vi "aquisicao.vi"(8 "Stop":bool, 9 "Number of Samples":i32=100, 10 "Sample Rate":dbl=1000.0, 11 "Physical Channel":tag="Dev1/ai0") -> (2 "Waveform Chart":waveform(dbl)(graph))   [LabVIEW 2019]
doc: "This example demonstrates how to continuously acquire buffered voltage measurements using a DAQmx device.\n\nFor instructions on how to connect your signals to the DAQ device, refer to your device documentation."
uses:
  <vilib>/Utility/error.llb/DialogType.ctl
  <vilib>/DAQmx/create/channels.llb/DAQmx Create Channel (AI-Voltage-Basic).vi
  <vilib>/DAQmx/configure/timing.llb/DAQmx Timing (Sample Clock).vi
  <vilib>/DAQmx/configure/task.llb/DAQmx Configure Logging (TDMS).vi
  <vilib>/DAQmx/miscellaneous.llb/DAQmx Fill In Error Info.vi
  <vilib>/DAQmx/read.llb/DAQmx Read (Analog Wfm 1Chan NSamp).vi
panel:
  in  "TDMS File Path":path
  in  "Logging Mode":i32(ring)=10231 items=["Off"=10231, "Log and Read"=15842]
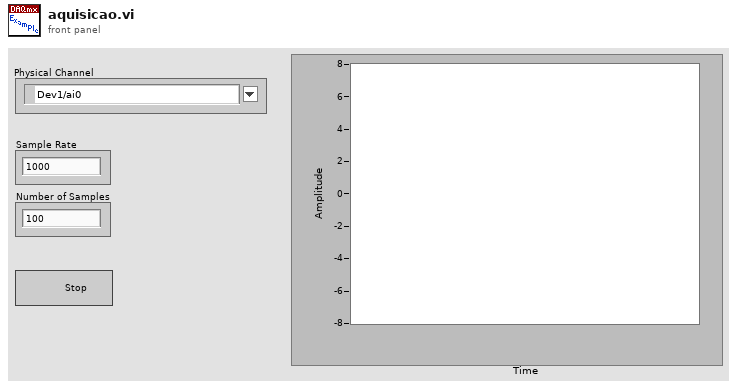
[diagram p1: front panel]
types:
  T1 = typedef "DialogType.ctl" = u16
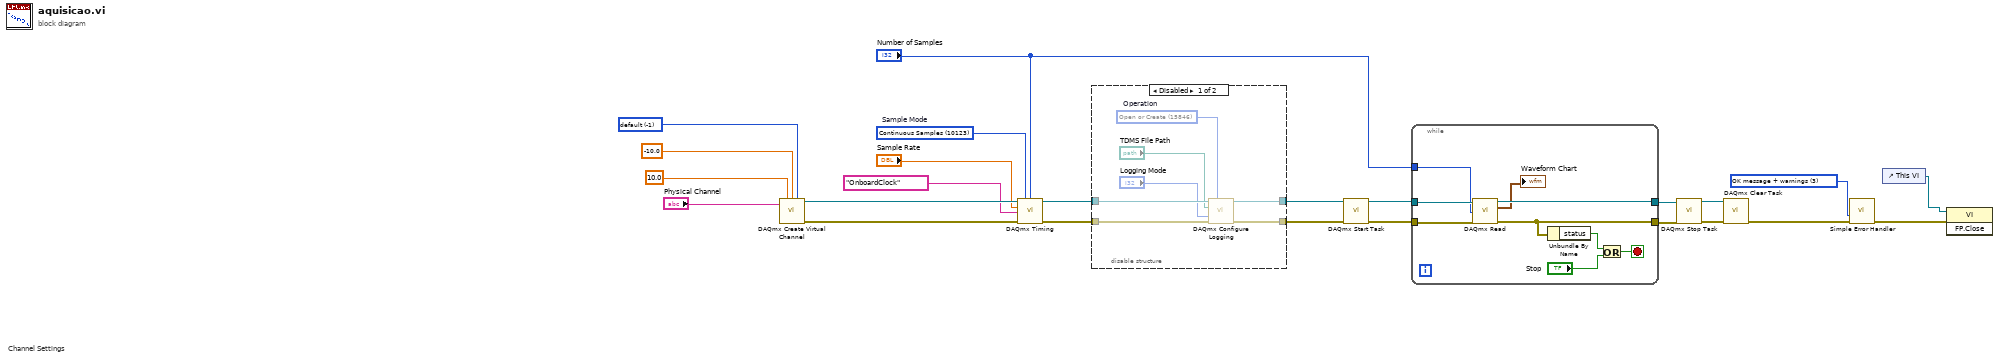
[diagram p0: block diagram]
diagram:
  w15 = -1 items=["default"=-1, "RSE"=10083, "NRSE"=10078, "Differential"=10106, "Pseudodifferential"=12529] ("Terminal Configuration")
  w5 = T1 3 items=["no dialog", "OK message", "continue or stop message", "OK message + warnings", "continue/stop + warnings"] ("type of dialog (OK msg:1)")
  w22 = 10123 items=["Finite Samples"=10178, "Continuous Samples"=10123, "Hardware Timed Single Point"=12522]  # Sample Mode
  # "Channel Settings"
  n1 = call-poly <vilib>:"DAQmx Create Virtual Channel.vi"("maximum value"=10.0 ("Max Voltage"), "minimum value"=-10.0 ("Min Voltage"), "input terminal configuration"=w15, "physical channels"="Physical Channel") -> ("task out"=w20:refnum<k21>, "error out"=w21:errorcluster)  [unwired: 10 in]
  n2 = call-poly <vilib>:"DAQmx Timing.vi"("task/channels in"=w20, "sample mode"=w22, "samples per channel"="Number of Samples", "rate"="Sample Rate", "source"=tag "OnboardClock" ("Sample Clock Source"), "error in"=w21) -> ("task out"=w24:refnum<k21>, "error out"=w23:errorcluster)  [unwired: 8 in]
  n3 = disable-structure shown="Disabled" {
    disable-tunnel: w24 -> [w31 w33]
    disable-tunnel: w23 -> [w30 w32]
    disable-tunnel: [w26 w33] -> w4
    disable-tunnel: [w25 w32] -> w3
    frame Disabled {
      w29 = 15846 items=["Open"=10437, "Open or Create"=15846, "Create or Replace"=15847, "Create"=15848]  # Operation
      n4 = call-poly <vilib>:"DAQmx Configure Logging.vi"("task/channels in"=w31, "operation"=w29, "file path"="TDMS File Path", "logging mode"="Logging Mode", "error in"=w30) -> ("task out"=w26:refnum<k21>, "error out"=w25:errorcluster)  [unwired: 9 in]
    }
    frame Enabled {
    }
  }
  n5 = call <vilib>:"DAQmx Start Task.vi"("task/channels in"=w4, "error in"=w3) -> ("task out"=w19:refnum<k21>, "error out"=w18:errorcluster)  [unwired: 12 in]
  n6 = while {
    tunnel: w19 -> [w42]
    tunnel: w18 -> [w41]
    tunnel: [w40] -> w9
    tunnel: [w37] -> w8
    tunnel: "Number of Samples" -> [w34]
    stop <- w35 stop-if-true
    n7 = call-poly <vilib>:"DAQmx Read.vi"("task/channels in"=w42, "number of samples per channel"=w34, "error in"=w41) -> ("task out"=w40:refnum<k21>, "data"=→"Waveform Chart":waveform(dbl), "error out"=w37:errorcluster)  [unwired: 10 in]
    n8 = Unbundle By Name(w37) -> ("status"=w36:bool)
    n9 = Or(x=w36, y="Stop") -> (x .or. y?=w35:bool)
  }
  n10 = call <vilib>:"DAQmx Stop Task.vi"("task/channels in"=w9, "error in"=w8) -> ("task out"=w6:refnum<k21>, "error out"=w7:errorcluster)  [unwired: 12 in]
  n11 = call <vilib>:"DAQmx Clear Task.vi"("task in"=w6, "error in"=w7) -> ("error out"=w17:errorcluster)  [unwired: 13 in]
  n12 = call <vilib>:"Simple Error Handler.vi"("type of dialog (OK msg:1)"=w5, "error in (no error)"=w17) -> ("error out"=w2:errorcluster)  [unwired: 3 in, 4 out]
  n13 = control-ref of="This VI"() -> (w1:refnum<vi>)
  n14 = invoke class="VI" method="FP.Close"(reference=w1, error in=w2) -> ()  [unwired: 1 in, 3 out]
